vi "Zwangsbedingungen.vi"(0 "AnzahlDIOs":i32, 1 "global stop RT":bool, 2 "Methodennummer":i32(ring) items=["0"], 3 "Mod1Mod2Mod3/AITrapsMachs1Hz":dbl[](array[numeric]), 4 "MWHorst":dbl[](array[numeric]), 5 "Zwangsbedingungen":dbl[][](array[numeric]), 6 "AnzahlLH":i32, 8 "AnzahlHorst":i32, 10 "AnzahlDIOs/Modul":i32[](array[numeric]), 12 "AnzahlHorst/Modul":i32[](array[numeric])) -> (7 "ZwangsFPGABoolesch?":bool[](array[boolean]), 9 "ZwangsFPGABoolesch!":bool[](array[boolean]), 11 "Methodennummer":i32(ring) items=["0"], 13 "global stop RT":bool, 14 "ZwangsDIO?":cluster{bool[]}[](array[cluster]), 15 "ZwangsDIO!":cluster{bool[]}[](array[cluster]), 16 "ZwangsLangsameH?":bool[](array[boolean]), 17 "ZwangsLangsameH!":bool[](array[boolean]), 18 "ZwangsHorst?":cluster{bool[]}[](array[cluster]), 19 "ZwangsHorst!":cluster{dbl[]}[](array[cluster]))   [LabVIEW 2010]
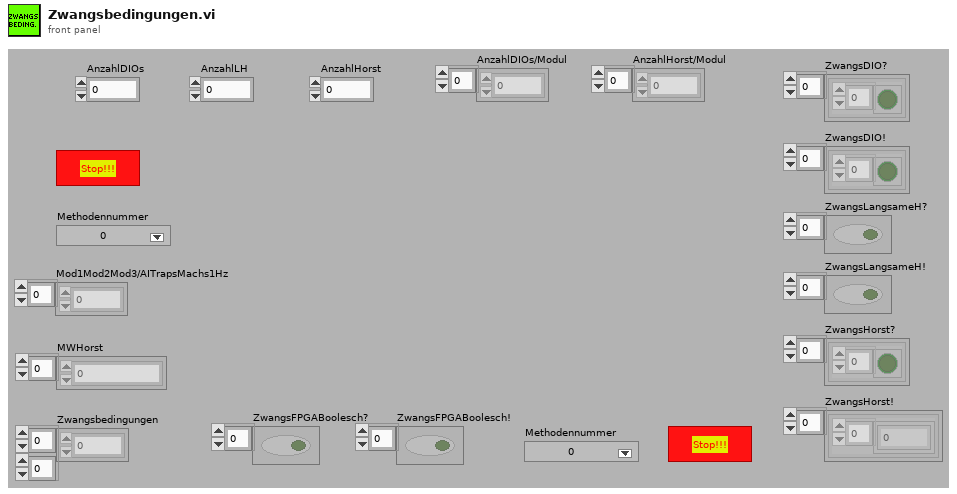
[diagram p1: front panel]
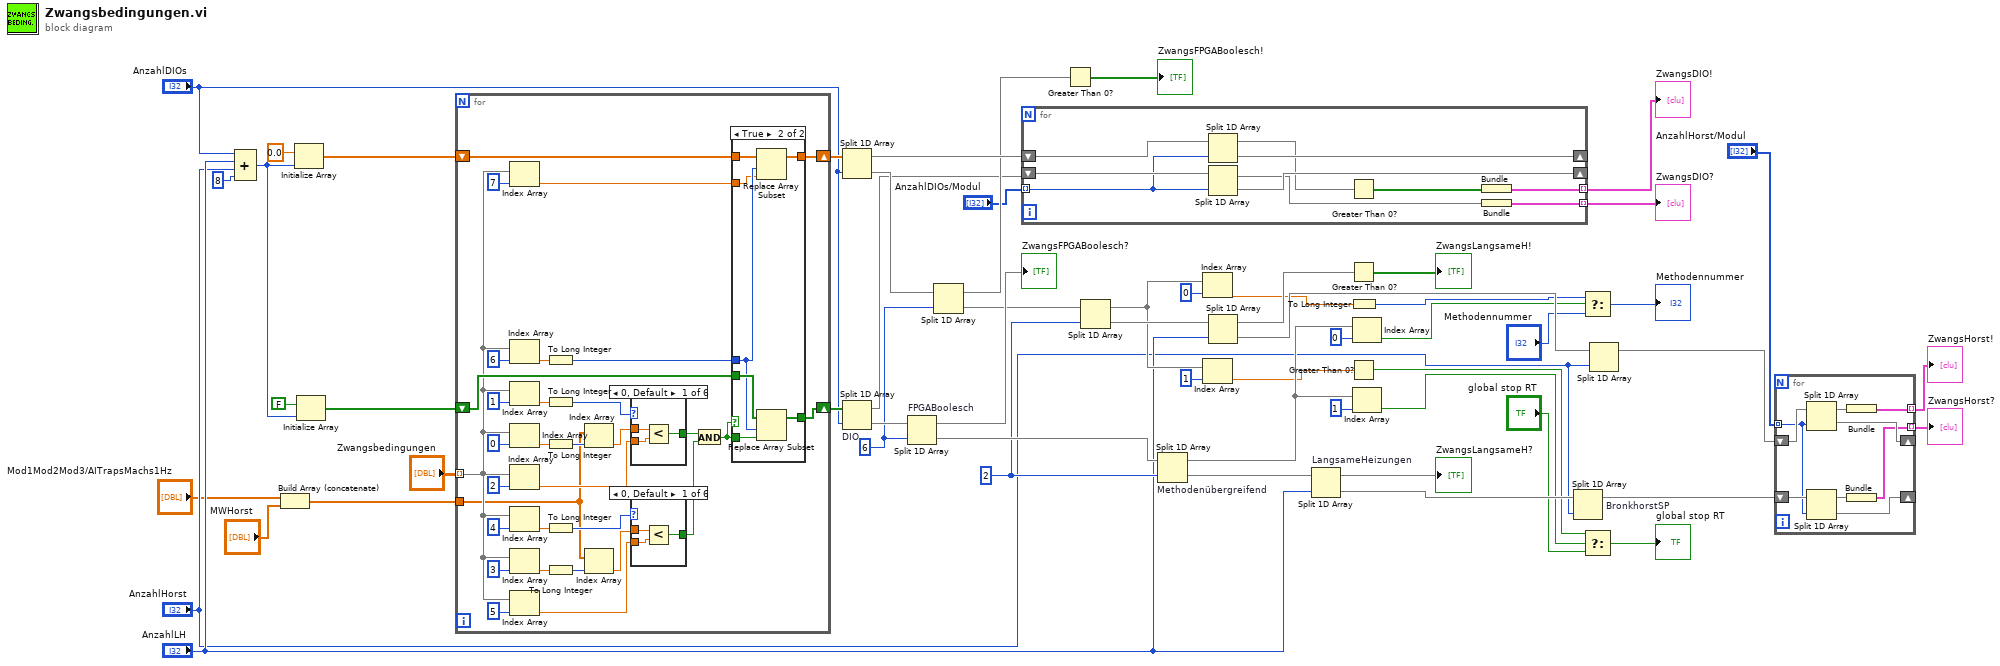
[diagram p0: block diagram]
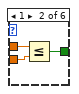
[diagram p2: hidden frame]
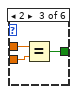
[diagram p3: hidden frame]
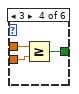
[diagram p4: hidden frame]
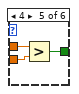
[diagram p5: hidden frame]
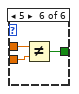
[diagram p6: hidden frame]
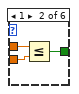
[diagram p8: hidden frame]
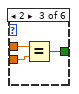
[diagram p9: hidden frame]
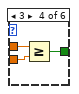
[diagram p10: hidden frame]
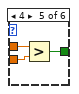
[diagram p11: hidden frame]
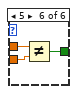
[diagram p12: hidden frame]
diagram:
  w36 = 2 ("Index")
  w50 = 6 ("Index")
  n1 = Compound Arithmetic op=ADD("AnzahlDIOs", "AnzahlLH", "AnzahlHorst", 8 ("Wert")) -> (w20:i32)
  n2 = Build Array (concatenate)("Mod1Mod2Mod3/AITrapsMachs1Hz", "MWHorst") -> (w57:dbl[])
  n3 = Initialize Array(0.0, w20) -> (w17:dbl[])
  n4 = Initialize Array(FALSE, w20) -> (w16:bool[])
  n5 = for {
    tunnel: w57 -> [w64]
    tunnel: "Zwangsbedingungen" -> [w68] mode=indexing
    shift-right: [w72] -> w56
    shift-left: w16 -> [w77]
    shift-right: [w73] -> w52
    shift-left: w17 -> [w76]
    n6 = Index Array(array=w68, index=7 ("Index")) -> (element=w74:dbl)
    n7 = Index Array(array=w68, index=6 ("Index")) -> (element=w79:dbl)
    n8 = Index Array(array=w68, index=1 ("Index")) -> (element=w86:dbl)
    n9 = Index Array(array=w68, index=0 ("Index")) -> (element=w88:dbl)
    n10 = Index Array(array=w68, index=2 ("Index")) -> (element=w82:dbl)
    n11 = Index Array(array=w68, index=4 ("Index")) -> (element=w62:dbl)
    n12 = Index Array(array=w68, index=3 ("Index")) -> (element=w63:dbl)
    n13 = Index Array(array=w68, index=5 ("Index")) -> (element=w61:dbl)
    n14 = To Long Integer(number=w79) -> (32bit integer=w75:i32)
    n15 = To Long Integer(number=w86) -> (32bit integer=w85:i32)
    n16 = To Long Integer(number=w88) -> (32bit integer=w81:i32)
    n17 = To Long Integer(number=w62) -> (32bit integer=w67:i32)
    n18 = To Long Integer(number=w63) -> (32bit integer=w65:i32)
    n19 = Index Array(array=w64, index=w81) -> (element=w84:dbl)
    n20 = Index Array(array=w64, index=w65) -> (element=w66:dbl)
    n21 = case shown="0, Default" w85 {
      tunnel: w84 -> [w119 w121 w125 w128 w131 w134]
      tunnel: w82 -> [w118 w122 w124 w127 w130 w133]
      tunnel: [w117 w120 w123 w126 w129 w132] -> w59
      frame 0, Default {
        n22 = Less?(x=w119, y=w118) -> (x < y?=w117:bool)
      }
      frame 1 {
        n23 = Less Or Equal?(x=w121, y=w122) -> (x <= y?=w120:bool)
      }
      frame 2 {
        n24 = Equal?(x=w125, y=w124) -> (x = y?=w123:bool)
      }
      frame 3 {
        n25 = Greater Or Equal?(x=w128, y=w127) -> (x >= y?=w126:bool)
      }
      frame 4 {
        n26 = Greater?(x=w131, y=w130) -> (0:w129:bool)
      }
      frame 5 {
        n27 = Not Equal?(x=w134, y=w133) -> (x != y?=w132:bool)
      }
    }
    n28 = case shown="0, Default" w67 {
      tunnel: w66 -> [w92 w94 w98 w101 w104 w107]
      tunnel: w61 -> [w91 w95 w97 w100 w103 w106]
      tunnel: [w90 w93 w96 w99 w102 w105] -> w60
      frame 0, Default {
        n29 = Less?(x=w92, y=w91) -> (x < y?=w90:bool)
      }
      frame 1 {
        n30 = Less Or Equal?(x=w94, y=w95) -> (x <= y?=w93:bool)
      }
      frame 2 {
        n31 = Equal?(x=w98, y=w97) -> (x = y?=w96:bool)
      }
      frame 3 {
        n32 = Greater Or Equal?(x=w101, y=w100) -> (x >= y?=w99:bool)
      }
      frame 4 {
        n33 = Greater?(x=w104, y=w103) -> (0:w102:bool)
      }
      frame 5 {
        n34 = Not Equal?(x=w107, y=w106) -> (x != y?=w105:bool)
      }
    }
    n35 = And(x=w59, y=w60) -> (x .and. y?=w58:bool)
    n36 = case shown="True" w58 {
      tunnel: w77 -> [w109 w116]
      tunnel: w76 -> [w108 w115]
      tunnel: w75 -> [_ w114]
      tunnel: w58 -> [_ w113]
      tunnel: w74 -> [_ w112]
      tunnel: [w108 w111] -> w73
      tunnel: [w109 w110] -> w72
      frame False {
      }
      frame True {
        n37 = Replace Array Subset(array=w115, new element=w112, index=w114) -> (w111:dbl[])
        n38 = Replace Array Subset(array=w116, new element=w113, index=w114) -> (w110:bool[])
      }
    }
  }
  n39 = Split 1D Array ("DIO")(array=w52, index="AnzahlDIOs") -> (first subarray=w51:dbl[], second subarray=w49:dbl[])
  n40 = Split 1D Array "DIO"(array=w56, index="AnzahlDIOs") -> (first subarray=w31:bool[], second subarray=w55:bool[])
  n41 = Split 1D Array "FPGABoolesch"(array=w55, index=w50) -> (first subarray=→"ZwangsFPGABoolesch?":bool[], second subarray=w40:bool[])
  n42 = Split 1D Array(array=w49, index=w50) -> (first subarray=w47:dbl[], second subarray=w38:dbl[])
  n43 = for {
    tunnel: [w137] -> w30 mode=indexing
    tunnel: "AnzahlDIOs/Modul" -> [w139] mode=indexing
    tunnel: [w135] -> w29 mode=indexing
    shift-right: [w143] -> _
    shift-left: w31 -> [w144]
    shift-right: [w141] -> _
    shift-left: w51 -> [w142]
    n44 = Split 1D Array(array=w142, index=w139) -> (first subarray=w140:dbl[], second subarray=w141:dbl[])
    n45 = Split 1D Array(array=w144, index=w139) -> (first subarray=w138:bool[], second subarray=w143:bool[])
    n46 = Greater Than 0?(x=w140) -> (x > 0?=w136:bool[])
    n47 = Bundle(w136) -> (w135:cluster{bool[]})  [unwired: 1 in]
    n48 = Bundle(w138) -> (w137:cluster{bool[]})  [unwired: 1 in]
  }
  "ZwangsDIO?" <- w30
  "ZwangsDIO!" <- w29
  n49 = Greater Than 0?(x=w47) -> (x > 0?=→"ZwangsFPGABoolesch!":bool[])
  n50 = Split 1D Array(array=w38, index=w36) -> (first subarray=w32:dbl[], second subarray=w37:dbl[])
  n51 = Split 1D Array "Methodenübergreifend"(array=w40, index=w36) -> (first subarray=w34:bool[], second subarray=w39:bool[])
  n52 = Index Array(array=w32, index=0 ("Index")) -> (element=w5:dbl)
  n53 = Index Array(array=w32, index=1 ("Index")) -> (element=w11:dbl)
  n54 = Split 1D Array(array=w37, index="AnzahlLH") -> (first subarray=w43:dbl[], second subarray=w45:dbl[])
  n55 = Split 1D Array "LangsameHeizungen"(array=w39, index="AnzahlLH") -> (first subarray=→"ZwangsLangsameH?":bool[], second subarray=w54:bool[])
  n56 = Greater Than 0?(x=w43) -> (x > 0?=→"ZwangsLangsameH!":bool[])
  n57 = To Long Integer(number=w5) -> (32bit integer=w3:i32)
  n58 = Greater Than 0?(x=w11) -> (x > 0?=w9:bool)
  n59 = Index Array(array=w34, index=0 ("Index")) -> (element=w4:bool)
  n60 = Index Array(array=w34, index=1 ("Index")) -> (element=w10:bool)
  n61 = Split 1D Array "BronkhorstSP"(array=w54, index="AnzahlHorst") -> (first subarray=w53:bool[])  [unwired: 1 out]
  n62 = Select(t=w3, s=w4, f="Methodennummer") -> (s? t:f=→"Methodennummer":i32)
  n63 = Select(t=w9, s=w10, f="global stop RT") -> (s? t:f=→"global stop RT":bool)
  n64 = Split 1D Array(array=w45, index="AnzahlHorst") -> (first subarray=w44:dbl[])  [unwired: 1 out]
  n65 = for {
    tunnel: "AnzahlHorst/Modul" -> [w150] mode=indexing
    shift-right: [w152] -> _
    shift-left: w53 -> [w153]
    tunnel: [w147] -> w28 mode=indexing
    shift-right: [w149] -> _
    shift-left: w44 -> [w151]
    tunnel: [w145] -> w27 mode=indexing
    n66 = Split 1D Array(array=w151, index=w150) -> (first subarray=w146:dbl[], second subarray=w149:dbl[])
    n67 = Split 1D Array(array=w153, index=w150) -> (first subarray=w148:bool[], second subarray=w152:bool[])
    n68 = Bundle(w146) -> (w145:cluster{dbl[]})  [unwired: 1 in]
    n69 = Bundle(w148) -> (w147:cluster{bool[]})  [unwired: 1 in]
  }
  "ZwangsHorst?" <- w28
  "ZwangsHorst!" <- w27
